vi "OPC UA Client-Write - Multiple Tags Example2.vi"() -> ()   [LabVIEW 2017]
uses:
  <vilib>/OPCUA/controls/NodeId.ctl
  <vilib>/OPCUA/controls/Write Status.ctl
  <vilib>/OPCUA/client/Multiple Write Double.vi
  <vilib>/OPCUA/NI OPC UA Client.lvlib
panel:
  in  "Array of NodeIds":string[](array[string])=["Process Data.Temperature1", "Process Data.Temperature2"]
  out "Temperature  Values":dbl[](array[numeric])=[25.343649970323533, 24.18860952393765]
  in  "Stop Button":bool
  in  "Server Endpoint URL":string="opc.tcp://XPS15HPH:49580"
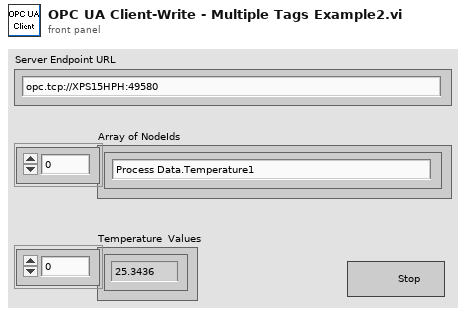
[diagram p1: front panel]
types:
  T1 = cluster{"message mode":enum16{"None", "Sign", "Sign and Encrypt"}, "security":enum16{"Basic256", "Basic128Rsa15"}}
  T2 = typedef "OPC UA Client Refnum.ctl" = refnum<k21>
  T3 = typedef "NodeId.ctl" = string
  T4 = typedef "Write Status.ctl" = u32
  T5 = cluster{"node ID":T3, "value":dbl, "timestamp (current time)":timestamp, "node status":T4}
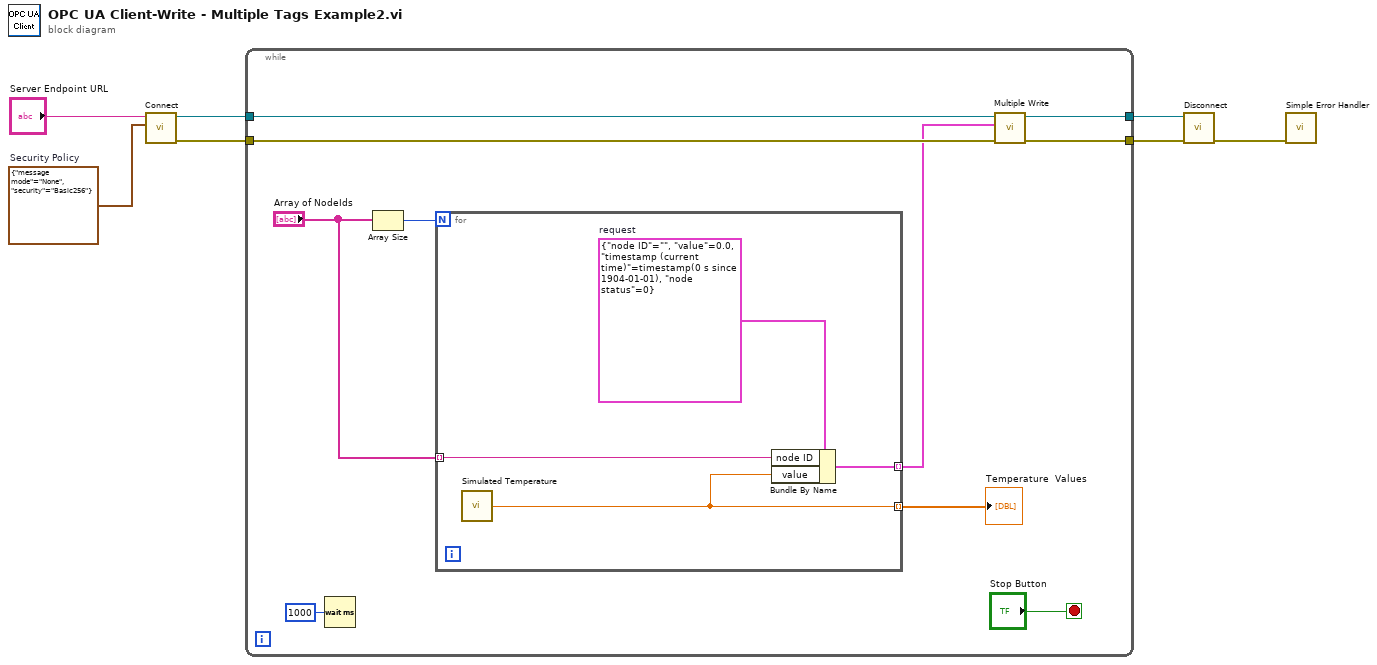
[diagram p0: block diagram]
diagram:
  w1 = T1 {"message mode"=enum."None", "security"=enum."Basic256"}  # Security Policy
  n1 = call <vilib>:"Connect.vi"("security policy"=w1, "server endpoint URL"="Server Endpoint URL") -> ("error out"=w6:errorcluster, "OPC UA client refnum out"=w7:T2)  [unwired: 7 in, 1 out]
  n2 = while {
    tunnel: w7 -> [w15]
    tunnel: w6 -> [w14]
    tunnel: [w13] -> w5
    tunnel: [w12] -> w3
    stop <- "Stop Button" stop-if-true
    n3 = Wait (ms)(milliseconds to wait=u32 1000) -> ()  [unwired: 1 out]
    n4 = Array Size(array="Array of NodeIds") -> (size(s)=w10:i32)
    n5 = for {
      N: w10 -> [_]
      tunnel: [w18] -> w11 mode=indexing
      tunnel: [w20] -> w9 mode=indexing
      tunnel: "Array of NodeIds" -> [w19] mode=indexing
      w21 = T5 {"node ID"="", "value"=0.0, "timestamp (current time)"=timestamp(0 s since 1904-01-01), "node status"=0}  # request
      n6 = call "Simulated Temperature.vi"() -> ("Temperature Value"=w18:dbl)  [unwired: 2 in]
      n7 = Bundle By Name(cluster=w21, "node ID"=w19, "value"=w18) -> (w20:T5)
    }
    "Temperature  Values" <- w11
    n8 = call-poly <vilib>:"Multiple Write.vi"("error in (no error)"=w14, "requests"=w9, "OPC UA client refnum in"=w15) -> ("error out"=w12:errorcluster, "OPC UA client refnum out"=w13:T2)  [unwired: 5 in, 2 out]
  }
  n9 = call <vilib>:"Disconnect.vi"("error in (no error)"=w3, "OPC UA client refnum in"=w5) -> ("error out"=w4:errorcluster)  [unwired: 9 in]
  n10 = call <vilib>:"Simple Error Handler.vi"("error in (no error)"=w4) -> ()  [unwired: 4 in, 5 out]
